vi "RegisterVI.vi"(8 "error in":errorcluster, 10 "VI Ref":refnum<vi>) -> (0 "error out":errorcluster, 1 "Current Language":string)   [LabVIEW 2020]
doc: "Register a VI to the localizer's registry. Automatically applies the current language to this VI."
uses:
  Localization FGV Action -- Enum.ctl
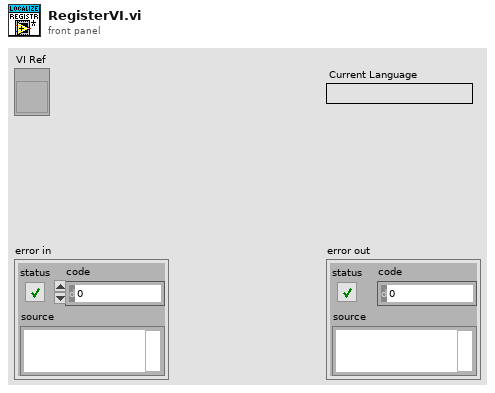
[diagram p1: front panel]
types:
  T1 = typedef "Localization FGV Action -- Enum.ctl" = enum16{"Read Dictionary", "Translate VIs", "Register VI", "Get Languages", "Translate Phrase", "Get Key For Phrase", "Get Phrase For Phrase", "Translate VI", "Unregister"}
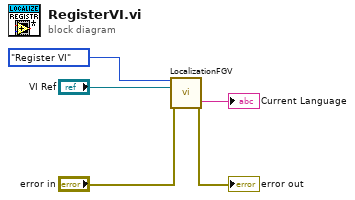
[diagram p0: block diagram]
diagram:
  n1 = call "LocalizationFGV.vi"("Action"=Localization_FGV_Action_--_Enum."Register VI", "VI in"="VI Ref", "error in"="error in") -> ("Current Language"=→"Current Language":string, "error out"=→"error out":errorcluster)  [unwired: 7 in, 4 out]
